vi "mainUIDisplayPython.vi"() -> ()   [LabVIEW 2017]
uses:
  globalUtilities.vi
  globalDevices.vi
panel:
  out "Numeric":i32
  in  "stop":bool
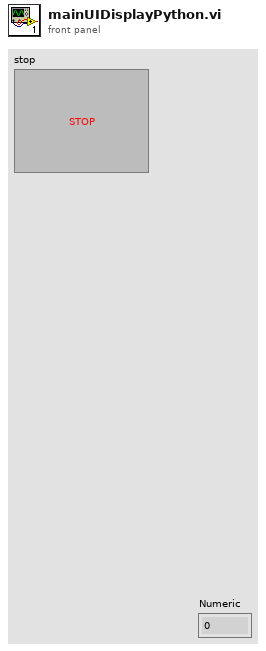
[diagram p1: front panel]
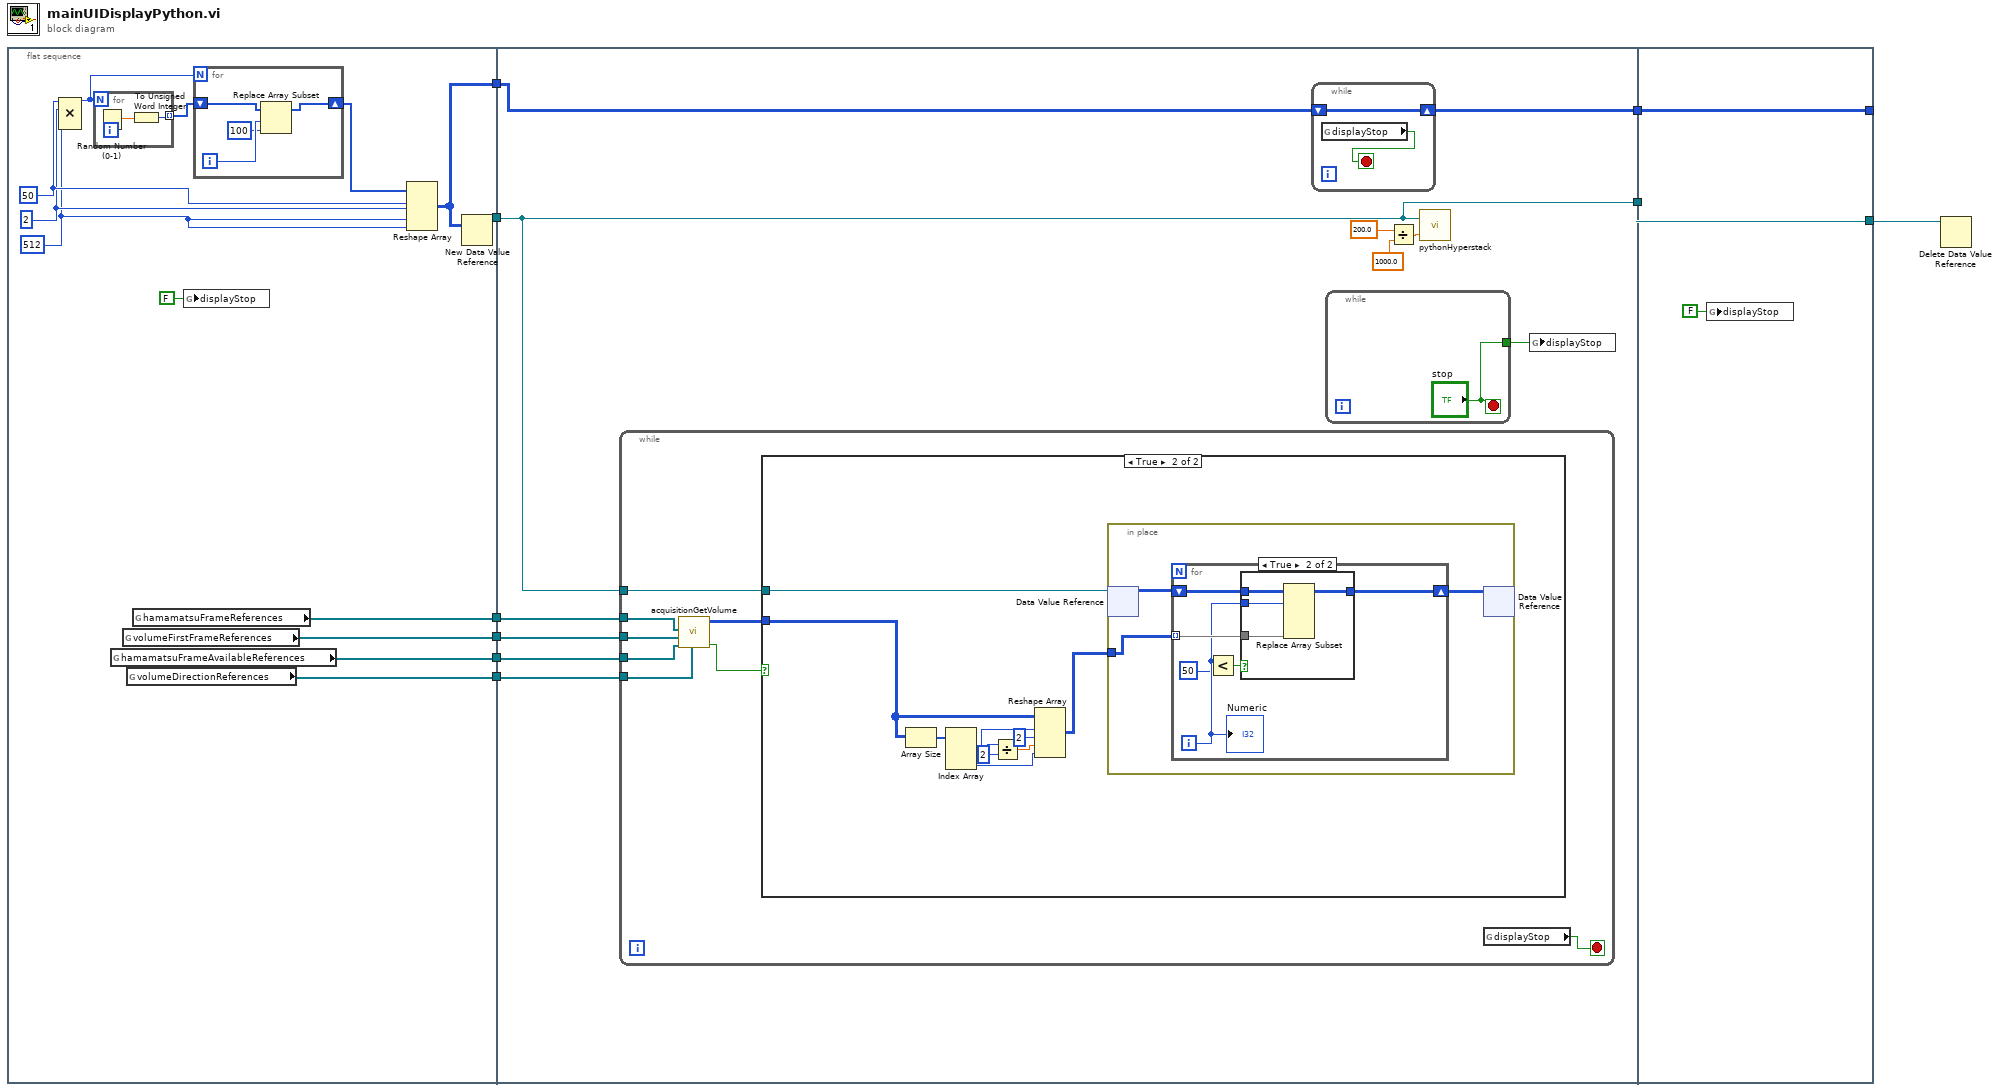
[diagram p0: block diagram]
diagram:
  n1 = flat-sequence {
    tunnel: [w19] -> w8
    tunnel: [w15] -> w7
    tunnel: [w13] -> w4
    tunnel: [w12] -> w3
    tunnel: [w11] -> w2
    tunnel: [w10] -> w1
    tunnel: w8 -> [w39]
    tunnel: [w38] -> w9
    tunnel: w7 -> [w33]
    tunnel: [w33] -> w6
    tunnel: w4 -> [w32]
    tunnel: w3 -> [w31]
    tunnel: w2 -> [w30]
    tunnel: w1 -> [w29]
    tunnel: w9 -> [w77]
    tunnel: [w77] -> _
    tunnel: w6 -> [w75]
    tunnel: [w75] -> w5
    frame #0 {
      w20 = 512 ("dimension size")
      w21 = 2 ("dimension size")
      w22 = 50 ("dimension size")
      n2 = Compound Arithmetic op=MULTIPLY(w22, w21, w20, w20) -> (w16:i32)
      n3 = for {
        N: w16 -> [_]
        tunnel: [w27] -> w18 mode=indexing
        n4 = Random Number (0-1)() -> (number: 0 to 1=w28:dbl)
        n5 = To Unsigned Word Integer(number=w28) -> (unsigned 16bit integer=w27:u16)
      }
      n6 = global read "globalDevices.vi" "hamamatsuFrameAvailableReferences"() -> (w11:refnum<data-value>[])
      n7 = global read "globalUtilities.vi" "volumeFirstFrameReferences"() -> (w12:refnum<data-value>[])
      n8 = global read "globalUtilities.vi" "volumeDirectionReferences"() -> (w10:refnum<data-value>[])
      n9 = global read "globalDevices.vi" "hamamatsuFrameReferences"() -> (w13:refnum<data-value>[])
      n10 = global write "globalUtilities.vi" "displayStop"(FALSE ("displayStop")) -> ()
      n11 = for {
        N: w16 -> [_]
        shift-right: [w23] -> w17
        shift-left: w18 -> [w26]
        i -> [w25]
        n12 = Replace Array Subset(array=w26, new element=u16 100 ("new element/subarray"), index=w25) -> (w23:u16[])
      }
      n13 = Reshape Array(w17, w22, w21, w20, w20) -> (w19:u16[][][][])
      n14 = New Data Value Reference(data value=w19) -> (data value reference=w15:refnum<data-value>)  [unwired: 1 in, 1 out]
    }
    frame #1 {
      n15 = while {
        tunnel: w33 -> [w47]
        tunnel: w32 -> [w46]
        tunnel: w31 -> [w45]
        tunnel: w30 -> [w44]
        tunnel: w29 -> [w43]
        stop <- w40 stop-if-true
        n16 = call "acquisitionGetVolume.vi"("volumeDirectionReferences"=w43, "hamamatsuFrameAvailableReferences"=w44, "volumeFirstFrameReferences"=w45, "hamamatsuFrameReferences"=w46) -> ("success"=w42:bool, "volume out"=w41:u16[][][])  [unwired: 1 in, 3 out]
        n17 = case shown="True" w42 {
          tunnel: w47 -> [_ w49]
          tunnel: w41 -> [_ w48]
          frame False {
          }
          frame True {
            n18 = Array Size(array=w48) -> (size(s)=w57:i32[])
            n19 = Index Array(array=w57) -> (element #1=w56:i32, element #2=w53:i32, element #3=w54:i32)  [unwired: 3 in]
            n20 = Divide(x=w53, y=2) -> (x/y=w51:dbl)
            n21 = Reshape Array(w48, w56, 2 ("dimension size"), w51, w54) -> (w50:u16[][][][])
            n22 = in-place {
              in-place-border: w50 -> [w59]
              n23 = in-place-dvr #1(w49) -> (w60:u16[][][][])  [unwired: 1 out]
              n24 = for {
                tunnel: w59 -> [w65] mode=indexing
                shift-right: [w64] -> w58
                shift-left: w60 -> [w66]
                i -> [w63]
                n25 = Less?(x=w63, y=50) -> (x < y?=w62:bool)
                n26 = case shown="True" w62 {
                  tunnel: w66 -> [w67 w71]
                  tunnel: w63 -> [_ w70]
                  tunnel: w65 -> [_ w69]
                  tunnel: [w67 w68] -> w64
                  frame False {
                  }
                  frame True {
                    n27 = Replace Array Subset(array=w71, new element=w69, index (dim 0)=w70) -> (w68:u16[][][][])  [unwired: 3 in]
                  }
                }
                "Numeric" <- w63
              }
              n28 = in-place-dvr #1(w58) -> ()  [unwired: 2 out]
            }
          }
        }
        n29 = global read "globalUtilities.vi" "displayStop"() -> (w40:bool)
      }
      n30 = while {
        shift-right: [w74] -> w38
        shift-left: w39 -> [w74]
        stop <- w73 stop-if-true
        n31 = global read "globalUtilities.vi" "displayStop"() -> (w73:bool)
      }
      n32 = while {
        tunnel: ["stop"] -> w34
        stop <- "stop" stop-if-true
      }
      n33 = Divide(x=200.0, y=1000.0) -> (x/y=w37:dbl)
      n34 = call "pythonHyperstack.vi"("refresh_time"=w37, "image reference"=w33) -> ()  [unwired: 1 out]
      n35 = global write "globalUtilities.vi" "displayStop"(w34) -> ()
    }
    frame #2 {
      n36 = global write "globalUtilities.vi" "displayStop"(FALSE ("displayStop")) -> ()
    }
  }
  n37 = Delete Data Value Reference(data value reference=w5) -> ()  [unwired: 1 in, 2 out]
